vi "JoystickDeadband.vi"(9 "DBPercent":dbl, 11 "JoystickIn":i32[](array[numeric])) -> (3 "JoystickOut":i32[](array[numeric]))   [LabVIEW 2013, in "ProcessorHelperFunctions.lvlib"]
uses:
  ProcessorHelperFunctions.lvlib
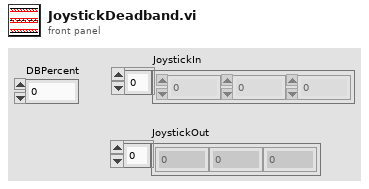
[diagram p1: front panel]
types:
  T1 = cluster{"JoystickIn[0]":i32, "JoystickIn[1]":i32, "JoystickIn[2]":i32, "JoystickIn[3]":i32, "JoystickIn[4]":i32, "JoystickIn[5]":i32, "JoystickIn[6]":i32, "JoystickIn[7]":i32, "JoystickIn[8]":i32, "JoystickIn[9]":i32}
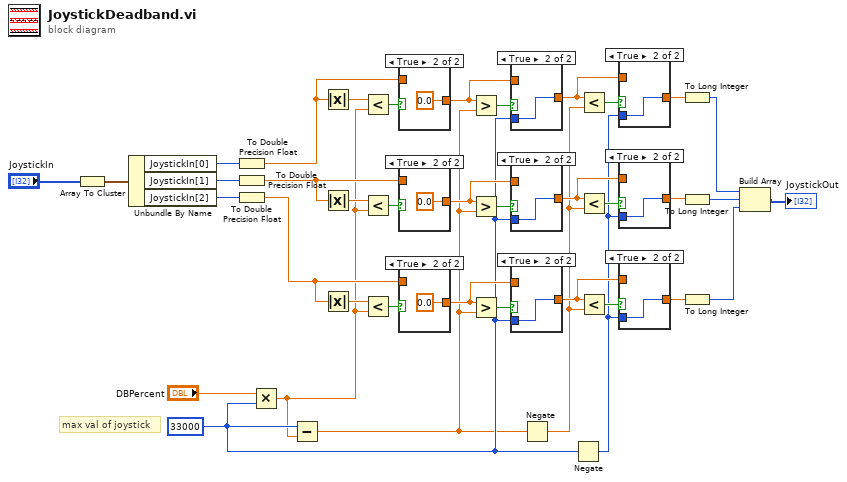
[diagram p0: block diagram]
diagram:
  w12 = 33000
  # "max val of joystick"
  n1 = Array To Cluster(array="JoystickIn") -> (cluster=w39:T1)
  n2 = Unbundle By Name(w39) -> ("JoystickIn[0]"=w35:i32, "JoystickIn[1]"=w28:i32, "JoystickIn[2]"=w27:i32)
  n3 = To Double Precision Float(number=w35) -> (double precision float=w29:dbl)
  n4 = To Double Precision Float(number=w28) -> (double precision float=w20:dbl)
  n5 = To Double Precision Float(number=w27) -> (double precision float=w13:dbl)
  n6 = Multiply(x="DBPercent", y=w12) -> (x*y=w8:dbl)
  n7 = Subtract(x=w12, y=w8) -> (x-y=w9:dbl)
  n8 = Absolute Value(x=w29) -> (abs(x)=w32:dbl)
  n9 = Absolute Value(x=w20) -> (abs(x)=w24:dbl)
  n10 = Absolute Value(x=w13) -> (abs(x)=w16:dbl)
  n11 = Less?(x=w32, y=w8) -> (x < y?=w36:bool)
  n12 = Less?(x=w24, y=w8) -> (x < y?=w21:bool)
  n13 = Less?(x=w16, y=w8) -> (x < y?=w19:bool)
  n14 = case shown="True" w36 {
    tunnel: w29 -> [w40 _]
    tunnel: [w40 0.0 ("JoystickIn[0]")] -> w33
    frame False {
    }
    frame True {
    }
  }
  n15 = case shown="True" w21 {
    tunnel: w20 -> [w42 _]
    tunnel: [w42 0.0 ("JoystickIn[0]")] -> w23
    frame False {
    }
    frame True {
    }
  }
  n16 = case shown="True" w19 {
    tunnel: w13 -> [w44 _]
    tunnel: [w44 0.0 ("JoystickIn[0]")] -> w17
    frame False {
    }
    frame True {
    }
  }
  n17 = Greater?(x=w33, y=w9) -> (0:w34:bool)
  n18 = Greater?(x=w23, y=w9) -> (0:w22:bool)
  n19 = Greater?(x=w17, y=w9) -> (0:w18:bool)
  n20 = case shown="True" w34 {
    tunnel: [w46 w47] -> w30
    tunnel: w33 -> [w46 _]
    tunnel: w12 -> [_ w47]
    frame False {
    }
    frame True {
    }
  }
  n21 = case shown="True" w22 {
    tunnel: [w48 w49] -> w26
    tunnel: w23 -> [w48 _]
    tunnel: w12 -> [_ w49]
    frame False {
    }
    frame True {
    }
  }
  n22 = case shown="True" w18 {
    tunnel: [w50 w51] -> w14
    tunnel: w17 -> [w50 _]
    tunnel: w12 -> [_ w51]
    frame False {
    }
    frame True {
    }
  }
  n23 = Negate(x=w9) -> (-x=w10:dbl)
  n24 = Negate(x=w12) -> (-x=w11:i32)
  n25 = Less?(x=w30, y=w10) -> (x < y?=w31:bool)
  n26 = Less?(x=w26, y=w10) -> (x < y?=w25:bool)
  n27 = Less?(x=w14, y=w10) -> (x < y?=w15:bool)
  n28 = case shown="True" w31 {
    tunnel: [w52 w53] -> w7
    tunnel: w30 -> [w52 _]
    tunnel: w11 -> [_ w53]
    frame False {
    }
    frame True {
    }
  }
  n29 = case shown="True" w25 {
    tunnel: [w54 w55] -> w6
    tunnel: w26 -> [w54 _]
    tunnel: w11 -> [_ w55]
    frame False {
    }
    frame True {
    }
  }
  n30 = case shown="True" w15 {
    tunnel: [w56 w57] -> w5
    tunnel: w14 -> [w56 _]
    tunnel: w11 -> [_ w57]
    frame False {
    }
    frame True {
    }
  }
  n31 = To Long Integer(number=w7) -> (32bit integer=w4:i32)
  n32 = To Long Integer(number=w6) -> (32bit integer=w3:i32)
  n33 = To Long Integer(number=w5) -> (32bit integer=w2:i32)
  n34 = Build Array(w4, w3, w2) -> (→"JoystickOut":i32[])
